vi "motor_test_oop_controller.vi"() -> ()   [LabVIEW 2019]
uses:
  MotorController.lvclass
  enable_disable_enum_typedef.ctl
  Axes_enum_typedef.ctl
panel:
  in  "Serial Port":refnum<visa-resource-name>
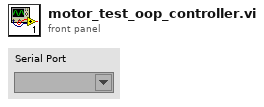
[diagram p1: front panel]
types:
  T1 = typedef "MotorController.lvclass/enable_disable_enum_typedef.ctl" = enum16{"Enable", "Disable"}
  T2 = typedef "Axes_enum_typedef.ctl" = enum16{"Polarizer 1", "Polarizer 2", "Sample", "Stage"}
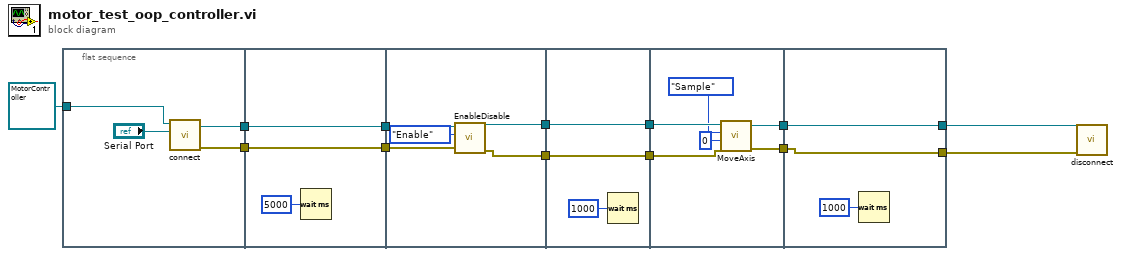
[diagram p0: block diagram]
diagram:
  n1 = flat-sequence {
    tunnel: refnum<class "MotorController.lvclass"> refnum ("MotorController.lvclass") -> [w16]
    tunnel: [w15] -> w12
    tunnel: [w14] -> w9
    tunnel: w12 -> [w19]
    tunnel: [w19] -> w11
    tunnel: [w18] -> w10
    tunnel: w9 -> [w18]
    tunnel: w11 -> [w25]
    tunnel: w10 -> [w24]
    tunnel: [w22] -> w8
    tunnel: [w21] -> w5
    tunnel: w8 -> [w27]
    tunnel: [w27] -> w7
    tunnel: [w26] -> w6
    tunnel: w5 -> [w26]
    tunnel: w7 -> [w34]
    tunnel: w6 -> [w31]
    tunnel: [w30] -> w4
    tunnel: [w29] -> w3
    tunnel: w4 -> [w36]
    tunnel: w3 -> [w35]
    tunnel: [w36] -> w2
    tunnel: [w35] -> w1
    frame #0 {
      n2 = call "connect.vi"("Serial Port"="Serial Port", "MotorController in"=w16) -> ("error out"=w14:errorcluster, "MotorController out"=w15:refnum<class "MotorController.lvclass">)  [unwired: 8 in]
    }
    frame #1 {
      n3 = Wait (ms)(milliseconds to wait=u32 5000) -> ()  [unwired: 1 out]
    }
    frame #2 {
      n4 = call "EnableDisable.vi"("error in (no error)"=w24, "Action"=enable_disable_enum_typedef."Enable", "MotorController in"=w25) -> ("error out"=w21:errorcluster, "MotorController out"=w22:refnum<class "MotorController.lvclass">)  [unwired: 7 in]
    }
    frame #3 {
      n5 = Wait (ms)(milliseconds to wait=u32 1000) -> ()  [unwired: 1 out]
    }
    frame #4 {
      n6 = call "MoveAxis.vi"("error in (no error)"=w31, "Position"=u16 0, "Axis"=Axes_enum_typedef."Sample", "MotorController in"=w34) -> ("error out"=w29:errorcluster, "MotorController out"=w30:refnum<class "MotorController.lvclass">)  [unwired: 6 in]
    }
    frame #5 {
      n7 = Wait (ms)(milliseconds to wait=u32 1000) -> ()  [unwired: 1 out]
    }
  }
  n8 = call "disconnect.vi"("error in (no error)"=w1, "MotorController in"=w2) -> ()  [unwired: 8 in, 2 out]
